vi "XNet Frame Id to Arb Id.vi"(11 "ID":u32) -> (3 "Arb id":u32)   [LabVIEW 2013, in "J1939.lvlib"]
uses:
  J1939.lvlib
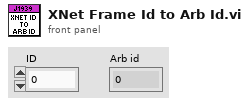
[diagram p1: front panel]
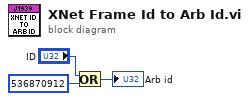
[diagram p0: block diagram]
diagram:
  n1 = Or(x="ID", y=u32 536870912) -> (x .or. y?=→"Arb id":u32)
